vi "Intensity Graph to Igor Graph.vi"(8 "error in (no error)":errorcluster, 9 "Filename":string="testname", 10 "Path":path=path "C:/temp", 11 "Intensity Graph Reference":refnum<vi>) -> (0 "error out":errorcluster, 2 "file":path)   [LabVIEW 2016, in "LVtoITX.lvclass"]
uses:
  LVtoITX.lvclass
  <userlib>/LevyLab/Graph Utilities/graph_utilities.lvclass/graph_utilities.ctl
  <userlib>/LevyLab/Graph Utilities/graph_utilities.lvclass
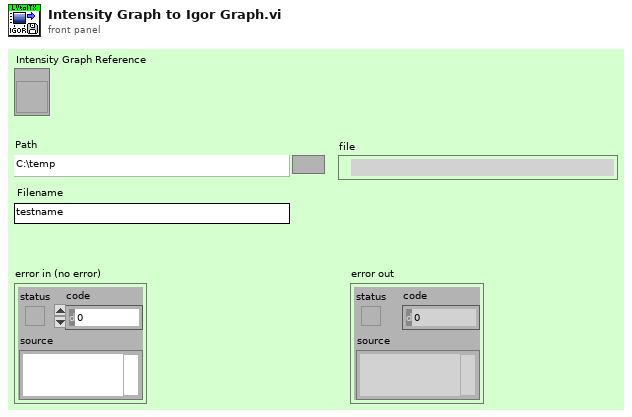
[diagram p1: front panel]
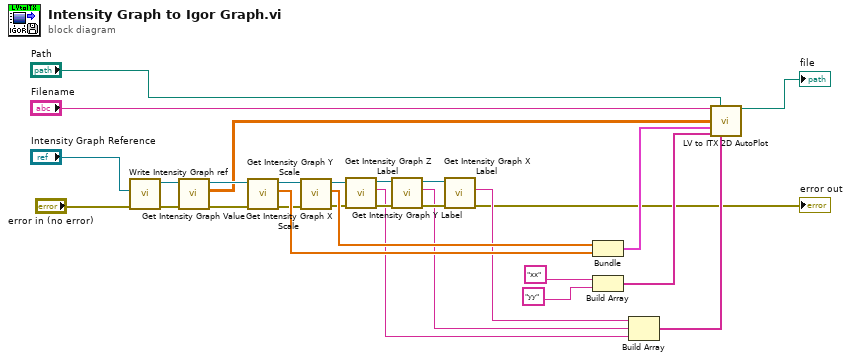
[diagram p0: block diagram]
diagram:
  n1 = call <userlib>:"Write Intensity Graph ref.vi"("error in (no error)"="error in (no error)", "Intensity Graph"="Intensity Graph Reference") -> ("error out"=w20:errorcluster, "graph_utilities out"=w21:refnum<class "graph_utilities.lvclass">)  [unwired: 8 in]
  n2 = call <userlib>:"Get Intensity Graph Value.vi"("error in (no error)"=w20, "graph_utilities in"=w21) -> ("error out"=w17:errorcluster, "Value"=w3:dbl[][], "graph_utilities out"=w18:refnum<class "graph_utilities.lvclass">)  [unwired: 7 in]
  n3 = call <userlib>:"Get Intensity Graph Y Scale.vi"("error in (no error)"=w17, "graph_utilities in"=w18) -> ("error out"=w14:errorcluster, "Y Scale"=w16:dbl[], "graph_utilities out"=w15:refnum<class "graph_utilities.lvclass">)  [unwired: 6 in, 1 out]
  n4 = call <userlib>:"Get Intensity Graph X Scale.vi"("error in (no error)"=w14, "graph_utilities in"=w15) -> ("error out"=w9:errorcluster, "X Scale"=w19:dbl[], "graph_utilities out"=w8:refnum<class "graph_utilities.lvclass">)  [unwired: 6 in, 1 out]
  n5 = call <userlib>:"Get Intensity Graph Z Label.vi"("error in (no error)"=w9, "graph_utilities in"=w8) -> ("error out"=w11:errorcluster, "Z Label"=w5:string, "graph_utilities out"=w10:refnum<class "graph_utilities.lvclass">)  [unwired: 7 in]
  n6 = call <userlib>:"Get Intensity Graph Y Label.vi"("error in (no error)"=w11, "graph_utilities in"=w10) -> ("error out"=w13:errorcluster, "Y Label"=w6:string, "graph_utilities out"=w12:refnum<class "graph_utilities.lvclass">)  [unwired: 7 in]
  n7 = call <userlib>:"Get Intensity Graph X Label.vi"("error in (no error)"=w13, "graph_utilities in"=w12) -> ("error out"=→"error out":errorcluster, "X Label"=w7:string)  [unwired: 7 in, 1 out]
  n8 = Bundle("X Scale"=w19, "Y Scale"=w16) -> (w26:cluster{"X Scale":dbl[], "Y Scale":dbl[]})  [unwired: 1 in]
  n9 = Build Array("xx" ("X Scale.Name Label.Text"), "yy" ("X Scale.Name Label.Text")) -> (w25:string[])
  n10 = Build Array(w7, w6, w5) -> (w27:string[])
  n11 = call "LV to ITX 2D AutoPlot.vi"("filename"="Filename", "path"="Path", "2D Array"=w3, "X, Y Arrays"=w26, "X, Y wavenames"=w25, "X,Y,Z Labels"=w27) -> ("file"=→"file":path)  [unwired: 9 in]
